vi "dashboard_to_read.vi"(1 "In":u8[](array[numeric])) -> (0 "Out":T1)   [LabVIEW 2022 SP3]
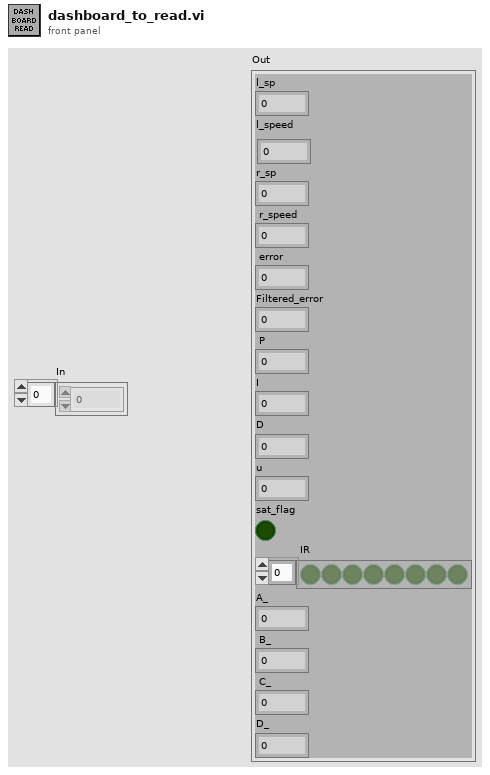
[diagram p1: front panel]
types:
  T1 = cluster{"l_sp":dbl, "l_speed":dbl, "r_sp":dbl, " r_speed":dbl, " error":dbl, "Filtered_error":dbl, " P":dbl, "I":dbl, "D":dbl, "u":dbl, "sat_flag":bool, " IR":bool[], "A_":dbl, " B_":dbl, " C_":dbl, "D_":dbl}
  T2 = cluster{i16, i16, i16, i16, i16, i16, i16, i16, i16, i16, u8, u8, i16, i16, i16, i16}
  T3 = cluster{"y":dbl, "y":dbl, "y":dbl, "y":dbl, "y":dbl, "y":dbl, "y":dbl, "y":dbl, "y":dbl, "y":dbl, bool, bool[], dbl, dbl, dbl, dbl}
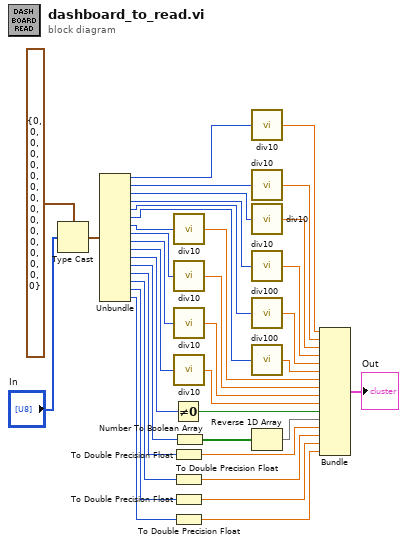
[diagram p0: block diagram]
diagram:
  n1 = Type Cast(type=T2 {0, 0, 0, 0, 0, 0, 0, 0, 0, 0, 0, 0, 0, 0, 0, 0}, x="In") -> (*(type *) &x=w35:T2)
  n2 = Unbundle(w35) -> (w34:i16, w33:i16, w32:i16, w31:i16, w30:i16, w29:i16, w28:i16, w27:i16, w26:i16, w25:i16, w24:u8, w23:u8, w21:i16, w20:i16, w19:i16, w18:i16)
  n3 = Not Equal To 0?(x=w24) -> (x != 0?=w7:bool)
  n4 = call "div10.vi"("x"=w28) -> ("y"=w11:dbl)
  n5 = call "div10.vi"("x"=w27) -> ("y"=w10:dbl)
  n6 = call "div10.vi"("x"=w26) -> ("y"=w9:dbl)
  n7 = call "div10.vi"("x"=w25) -> ("y"=w8:dbl)
  n8 = To Double Precision Float(number=w21) -> (double precision float=w6:dbl)
  n9 = To Double Precision Float(number=w20) -> (double precision float=w5:dbl)
  n10 = To Double Precision Float(number=w19) -> (double precision float=w4:dbl)
  n11 = To Double Precision Float(number=w18) -> (double precision float=w3:dbl)
  n12 = Number To Boolean Array(number=w23) -> (Boolean array=w2:bool[])
  n13 = call "div10.vi"("x"=w34) -> ("y"=w22:dbl)
  n14 = call "div10.vi"("x"=w33) -> ("y"=w16:dbl)
  n15 = call "div10.vi"("x"=w32) -> ("y"=w15:dbl)
  n16 = call "div10.vi"("x"=w31) -> ("y"=w14:dbl)
  n17 = call "div100.vi"("x"=w30) -> ("y"=w13:dbl)
  n18 = call "div100.vi"("x"=w29) -> ("y"=w12:dbl)
  n19 = Reverse 1D Array(array=w2) -> (reversed array=w1:bool[])
  n20 = Bundle("y"=w22, "y"=w16, "y"=w15, "y"=w14, "y"=w13, "y"=w12, "y"=w11, "y"=w10, "y"=w9, "y"=w8, w7, w1, w6, w5, w4, w3) -> (→"Out":T3)  [unwired: 1 in]
